vi "Execute.vi"(8 "error in (no error)":errorcluster, 11 "iProcess Step Model in":refnum<class "iProcess Step Model.lvclass">) -> (0 "error out":errorcluster, 3 "iProcess Step Model out":refnum<class "iProcess Step Model.lvclass">)   [LabVIEW 2017, in "iProcess Step Model.lvlib" / "iProcess Step Model.lvclass"]
uses:
  iProcess Step Model.lvclass
  C:/Program Files/National Instruments/LabVIEW 2017/vi.lib/ActorFramework/Actor/Actor.lvclass
  <vilib>/ActorFramework/Actor/Actor.lvclass/Actor.ctl
  <vilib>/ActorFramework/Message Enqueuer/Message Enqueuer.lvclass/Message Enqueuer.ctl
  <vilib>/ActorFramework/Message Enqueuer/Init from Existing Queue.vi
  <vilib>/ActorFramework/Message Enqueuer/Enqueue.vi
  iProcess Step Model Messages/Execute Msg/Execute Msg.lvclass
  C:/Program Files/National Instruments/LabVIEW 2017/vi.lib/ActorFramework/Message/Message.lvclass
  <vilib>/ActorFramework/Message Priority Queue/Priority Enqueue.vi
  <vilib>/ActorFramework/Message Enqueuer/Message Enqueuer.lvclass
  <vilib>/ActorFramework/Actor/Actor.lvclass
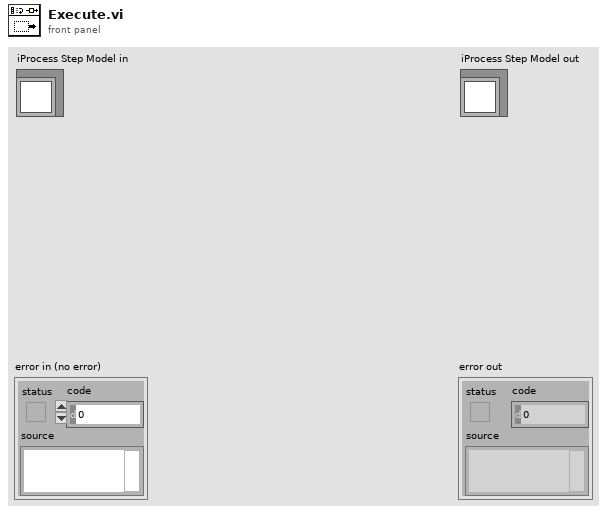
[diagram p1: front panel]
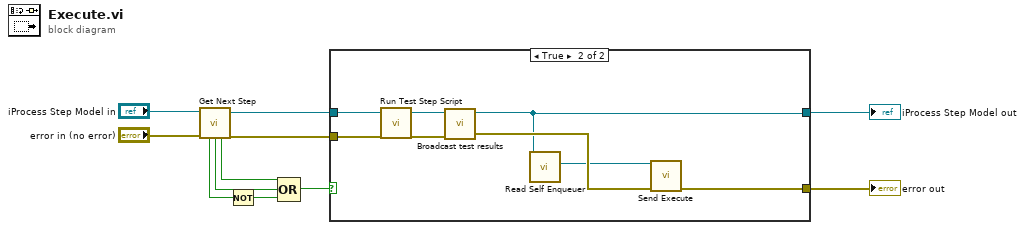
[diagram p0: block diagram]
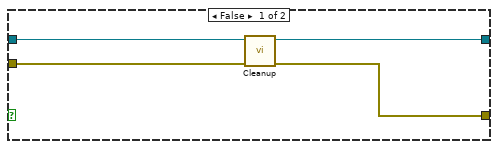
[diagram p2: hidden frame]
diagram:
  n1 = call-dynamic "Get Next Step.vi"("iProcess Step Model in"="iProcess Step Model in", "error in (no error)"="error in (no error)") -> ("iProcess Step Model out"=w9:refnum<class "iProcess Step Model.lvclass">, "Found"=w8:bool, "Complete"=w6:bool, "Stop"=w7:bool, "error out"=w4:errorcluster)  [unwired: 9 in]
  n2 = Not(x=w8) -> (.not. x?=w5:bool)
  n3 = Compound Arithmetic op=OR(w7, w6, w5) -> (w1:bool)
  n4 = case shown="True" w1 {
    tunnel: w9 -> [w15 w23]
    tunnel: w4 -> [w14 w20]
    tunnel: [w13 w18] -> w3
    tunnel: [w12 w17] -> w2
    frame False {
      n5 = call-dynamic "Cleanup.vi"("error in (no error)"=w14, "iProcess Step Model in"=w15) -> ("error out"=w13:errorcluster, "iProcess Step Model out"=w12:refnum<class "iProcess Step Model.lvclass">)  [unwired: 8 in]
    }
    frame True {
      n6 = call-dynamic "Run Test Step Script.vi"("error in (no error)"=w20, "iProcess Step Model in"=w23) -> ("error out"=w21:errorcluster, "iProcess Step Model out"=w22:refnum<class "iProcess Step Model.lvclass">)  [unwired: 8 in]
      n7 = call-dynamic "Broadcast test results.vi"("error in (no error)"=w21, "iProcess Step Model in"=w22) -> ("error out"=w19:errorcluster, "iProcess Step Model out"=w17:refnum<class "iProcess Step Model.lvclass">)  [unwired: 8 in]
      n8 = call <vilib>:"Read Self Enqueuer.vi"("Actor"=w17) -> ("Self Enqueuer"=w16:refnum<class "Message Enqueuer.lvclass">)  [unwired: 10 in]
      n9 = call "Send Execute.vi"("error in (no error)"=w19, "Message Enqueuer"=w16) -> ("error out"=w18:errorcluster)  [unwired: 8 in, 1 out]
    }
  }
  "error out" <- w3
  "iProcess Step Model out" <- w2
